vi "Main 9626.vi"() -> ()   [LabVIEW 2014]
uses:
  <vilib>/rvi/Emulation/niFpgaGetClockAttributes.vi
  <vilib>/rvi/Emulation/niFpgaSctlEmulationGetInTimedLoop.vi
  <vilib>/rvi/Emulation/niFpgaEmulationReportErrorSimple.vi
  <vilib>/rvi/eio/common/nirviEmuTemplateMethod_errors.vi
  <vilib>/rvi/Emulation/niFpgaCriticalErrorInLSC.vi
  <vilib>/eio/EIOMethodNode/EIOMethodNode.xnode
panel:
  out "RMC/DIO 0":bool
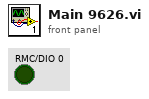
[diagram p1: front panel]
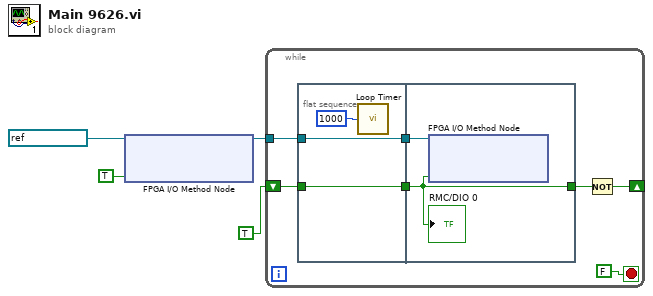
[diagram p0: block diagram]
diagram:
  n1 = xnode "FPGA I/O Method Node"("FPGA I/O In"=refnum<k21> "RMC/DIO0", "Enable"=TRUE) -> ("FPGA I/O Out"=w2:refnum<k21>)
  n2 = while {
    shift-right: [w8] -> _
    shift-left: TRUE -> [w10]
    tunnel: w2 -> [w5]
    stop <- FALSE stop-if-true
    n3 = flat-sequence {
      tunnel: w10 -> [w13]
      tunnel: [w13] -> w9
      tunnel: w5 -> [w12]
      tunnel: [w12] -> w6
      tunnel: w9 -> [w16]
      tunnel: [w16] -> w7
      tunnel: w6 -> [w15]
      frame #0 {
        n4 = call "Loop Timer"("Count(mSec)"=u32 1000) -> ()  [unwired: 1 out]
      }
      frame #1 {
        n5 = xnode "FPGA I/O Method Node"("FPGA I/O In"=w15, "Data"=w16) -> ()  [unwired: 1 out]
        "RMC/DIO 0" <- w16
      }
    }
    n6 = Not(x=w7) -> (.not. x?=w8:bool)
  }
